vi "Numeric_Integer_Operations.vi"() -> ()   [LabVIEW 2019]
panel:
  out "Numeric 8":i64
  in  "Numeric 7":i64
  out "Numeric 6":i16
  in  "Numeric 5":i16
  out "Numeric 4":u8
  in  "Numeric 3":u8
  out "Numeric 2":i8
  in  "Numeric":i8
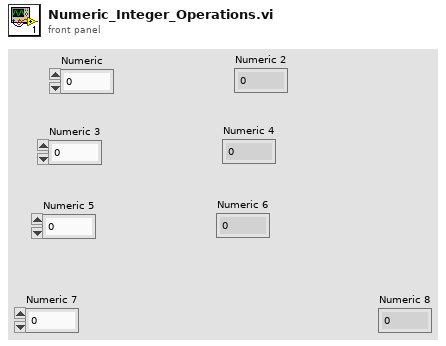
[diagram p1: front panel]
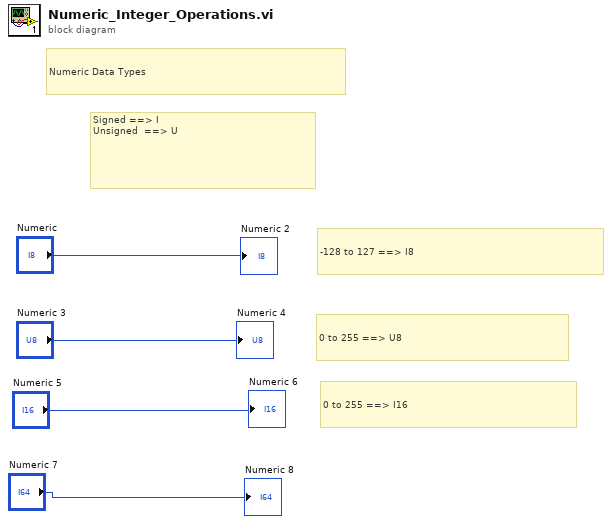
[diagram p0: block diagram]
diagram:
  # "0 to 255 ==> I16"
  # "0 to 255 ==> U8"
  # "-128 to 127 ==> I8"
  # "Signed ==> I\nUnsigned  ==> U"
  # "Numeric Data Types"
  "Numeric 2" <- "Numeric"
  "Numeric 4" <- "Numeric 3"
  "Numeric 6" <- "Numeric 5"
  "Numeric 8" <- "Numeric 7"
